vi "多合一臂环解析.vi"(11 "数组":u8[](array[numeric])) -> (0 "chn6":i32(graph), 1 "chn3":i32(graph), 2 "chn8":i32(graph), 3 "chn1":i32(graph), 4 "chn7":i32(graph), 5 "chn2":i32(graph), 6 "chn4":i32(graph), 7 "chn5":i32(graph))   [LabVIEW 2023]
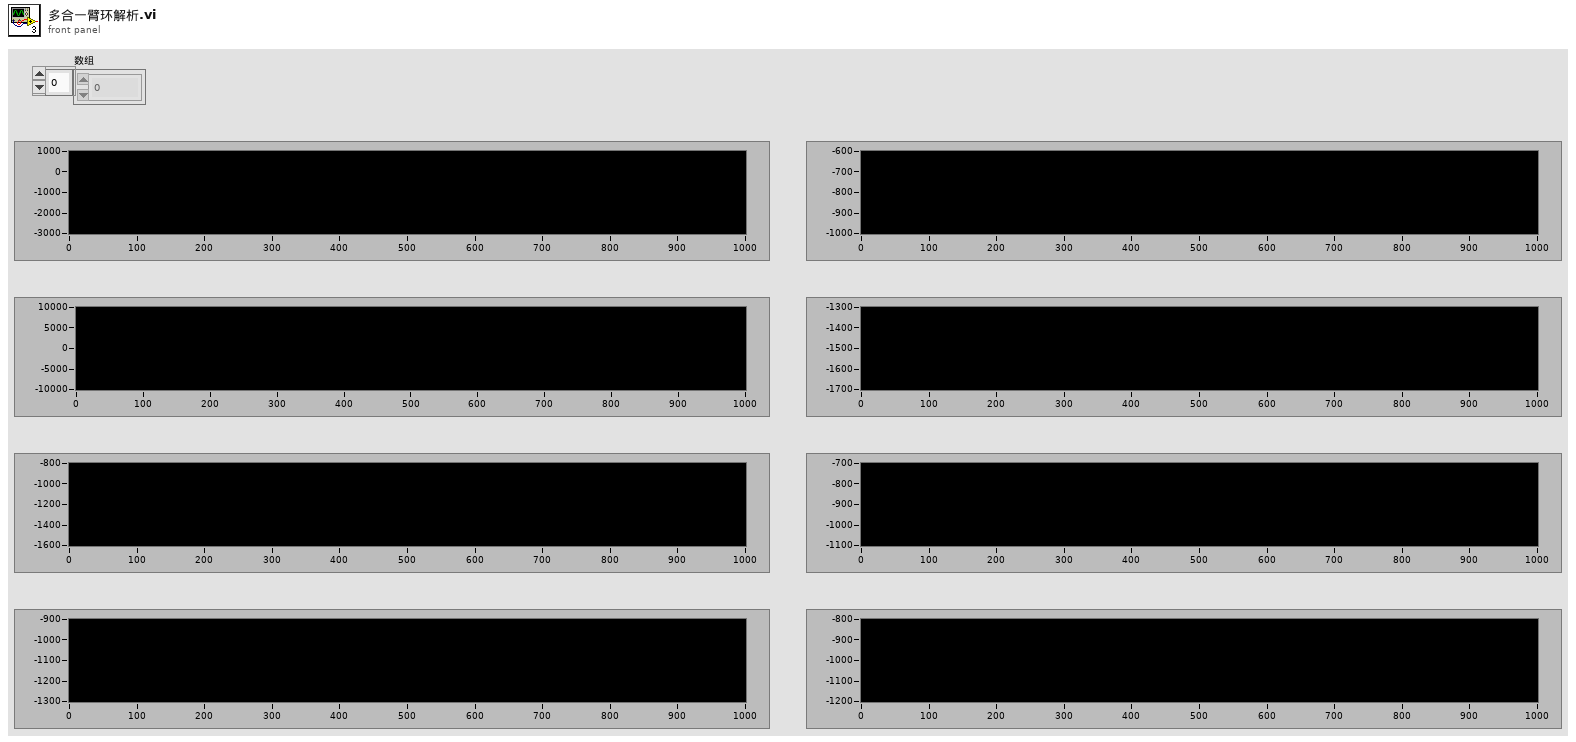
[diagram p1: front panel]
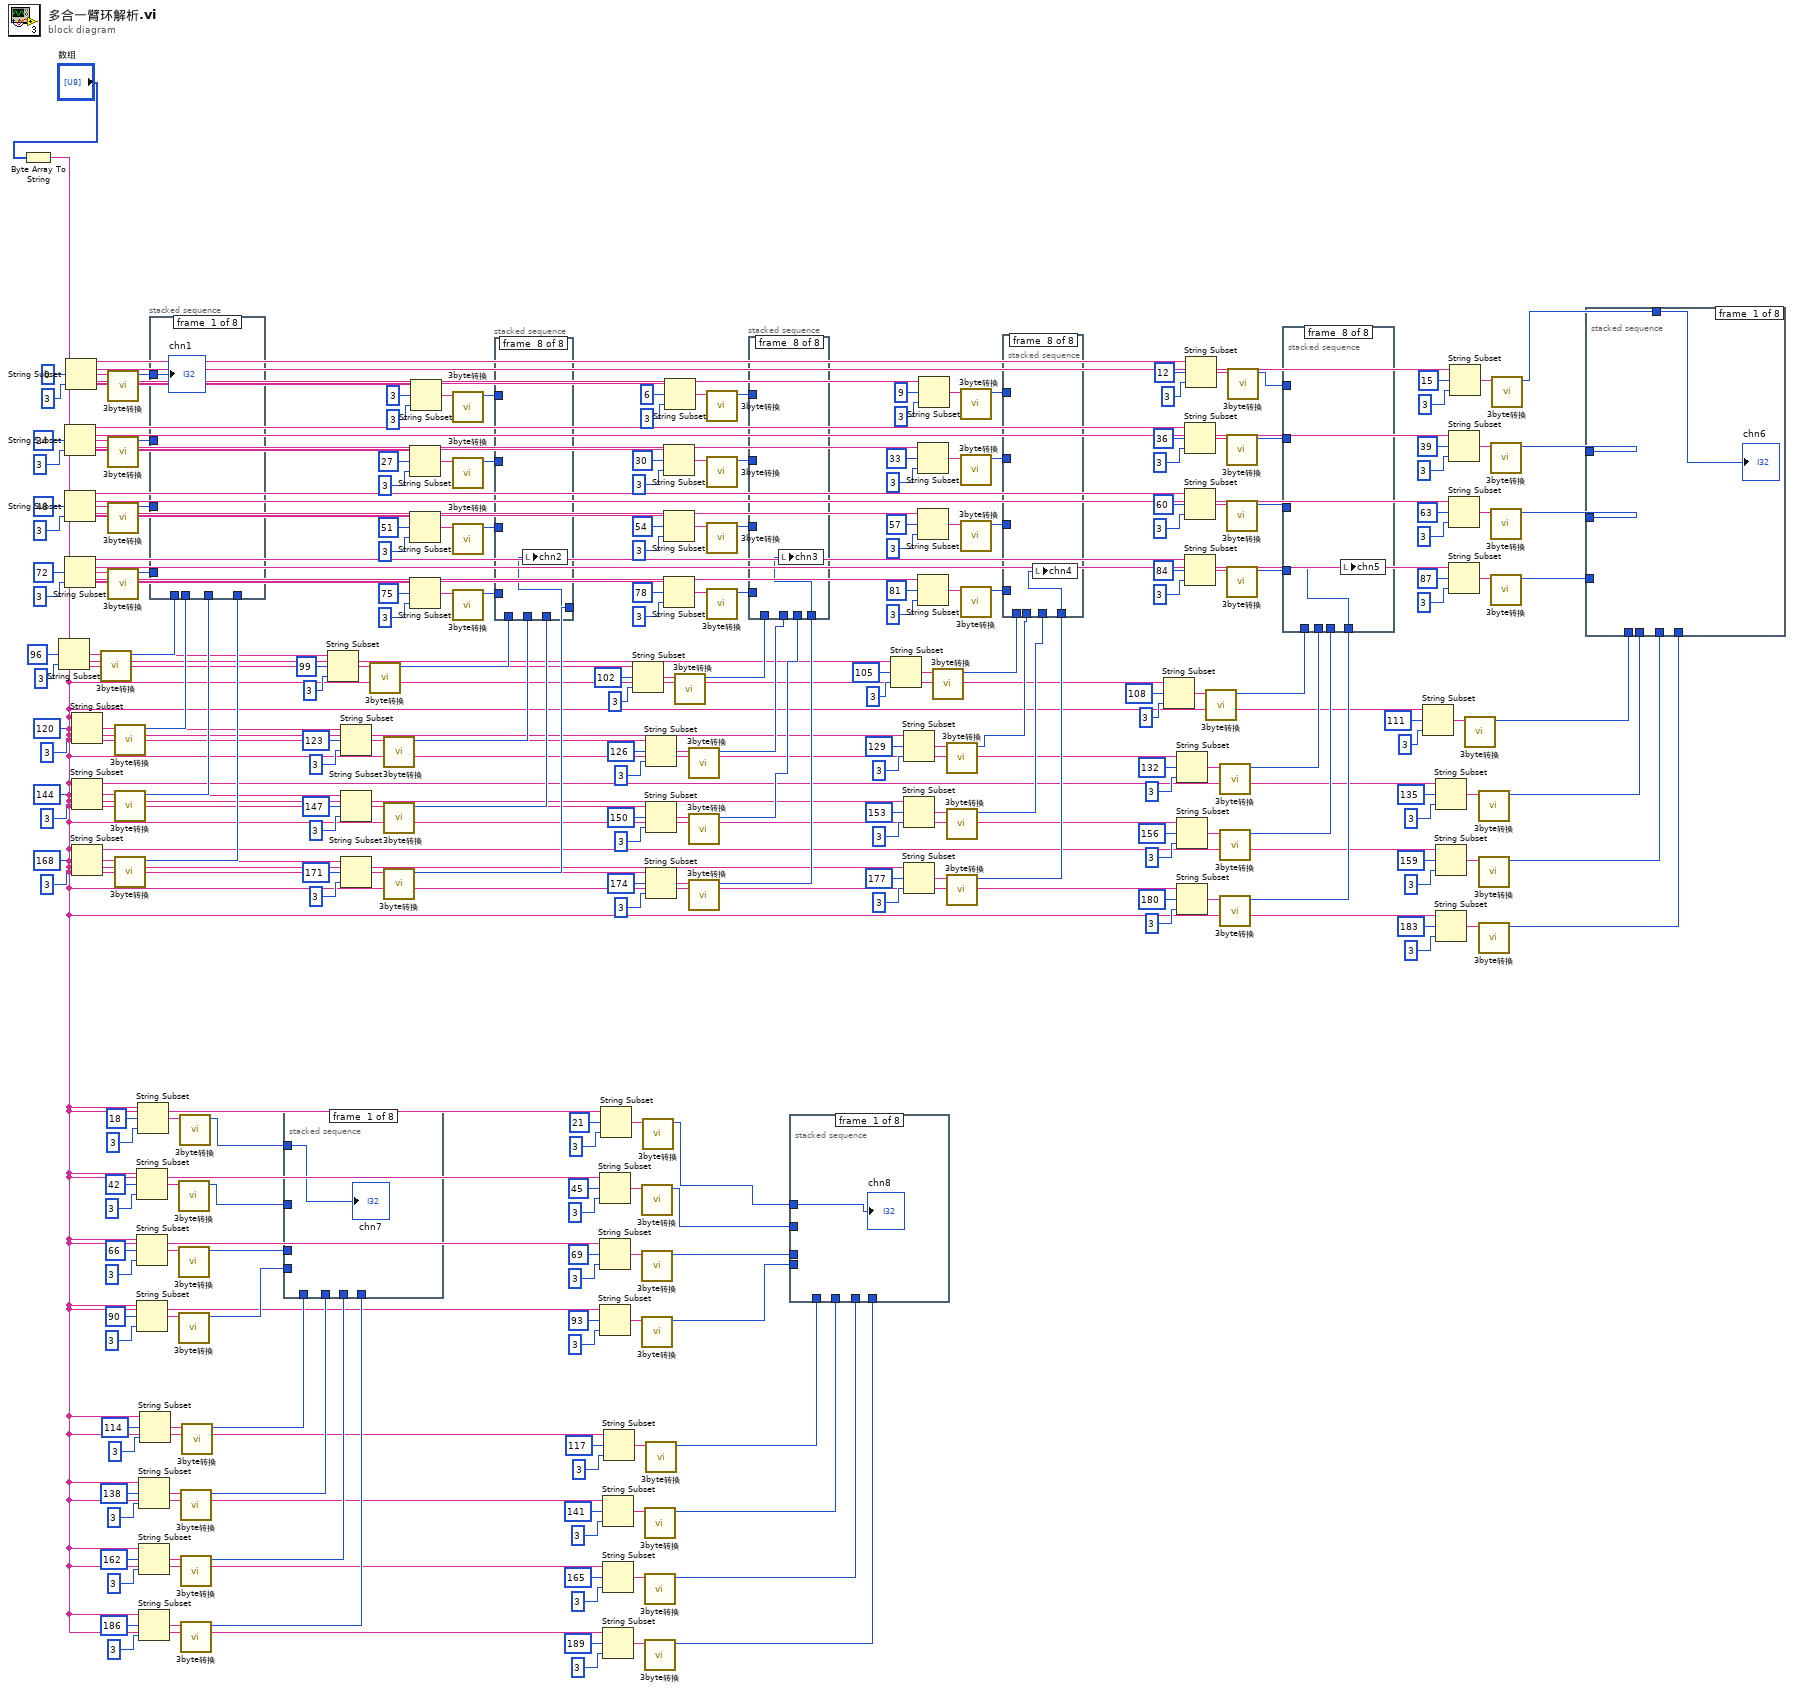
[diagram p0: block diagram]
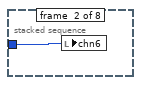
[diagram p2: hidden frame]
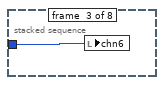
[diagram p3: hidden frame]
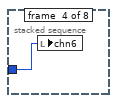
[diagram p4: hidden frame]
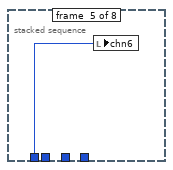
[diagram p5: hidden frame]
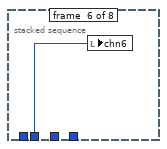
[diagram p6: hidden frame]
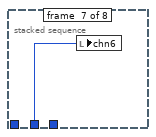
[diagram p7: hidden frame]
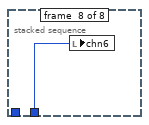
[diagram p8: hidden frame]
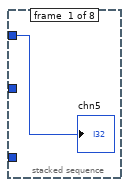
[diagram p9: hidden frame]
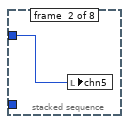
[diagram p10: hidden frame]
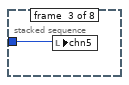
[diagram p11: hidden frame]
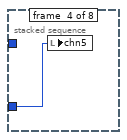
[diagram p12: hidden frame]
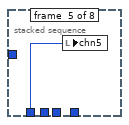
[diagram p13: hidden frame]
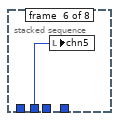
[diagram p14: hidden frame]
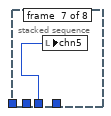
[diagram p15: hidden frame]
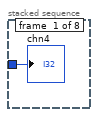
[diagram p16: hidden frame]
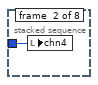
[diagram p17: hidden frame]
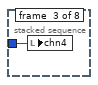
[diagram p18: hidden frame]
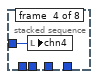
[diagram p19: hidden frame]
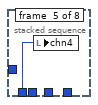
[diagram p20: hidden frame]
diagram:
  n1 = Byte Array To String(unsigned byte array="数组") -> (string=w5:string)
  n2 = String Subset(string=w5, offset (0)=96 ("偏移量(0)"), length (rest)=3 ("长度（剩余）")) -> (substring=w129:string)
  n3 = String Subset(string=w5, offset (0)=24 ("偏移量(0)"), length (rest)=3 ("长度（剩余）")) -> (substring=w256:string)
  n4 = String Subset(string=w5, offset (0)=48 ("偏移量(0)"), length (rest)=3 ("长度（剩余）")) -> (substring=w255:string)
  n5 = String Subset(string=w5, offset (0)=72 ("偏移量(0)"), length (rest)=3 ("长度（剩余）")) -> (substring=w254:string)
  n6 = String Subset(string=w5, offset (0)=0 ("偏移量(0)"), length (rest)=3 ("长度（剩余）")) -> (substring=w257:string)
  n7 = String Subset(string=w5, offset (0)=120 ("偏移量(0)"), length (rest)=3 ("长度（剩余）")) -> (substring=w128:string)
  n8 = String Subset(string=w5, offset (0)=144 ("偏移量(0)"), length (rest)=3 ("长度（剩余）")) -> (substring=w127:string)
  n9 = String Subset(string=w5, offset (0)=168 ("偏移量(0)"), length (rest)=3 ("长度（剩余）")) -> (substring=w126:string)
  n10 = call "3byte转换.vi"("字符串"=w129) -> ("数值"=w118:i32)  [unwired: 10 in]
  n11 = call "3byte转换.vi"("字符串"=w257) -> ("数值"=w245:i32)  [unwired: 10 in]
  n12 = call "3byte转换.vi"("字符串"=w256) -> ("数值"=w244:i32)  [unwired: 10 in]
  n13 = call "3byte转换.vi"("字符串"=w255) -> ("数值"=w243:i32)  [unwired: 10 in]
  n14 = call "3byte转换.vi"("字符串"=w254) -> ("数值"=w242:i32)  [unwired: 10 in]
  n15 = call "3byte转换.vi"("字符串"=w128) -> ("数值"=w117:i32)  [unwired: 10 in]
  n16 = call "3byte转换.vi"("字符串"=w127) -> ("数值"=w116:i32)  [unwired: 10 in]
  n17 = call "3byte转换.vi"("字符串"=w126) -> ("数值"=w115:i32)  [unwired: 10 in]
  n18 = String Subset(string=w5, offset (0)=42 ("偏移量(0)"), length (rest)=3 ("长度（剩余）")) -> (substring=w160:string)
  n19 = String Subset(string=w5, offset (0)=66 ("偏移量(0)"), length (rest)=3 ("长度（剩余）")) -> (substring=w159:string)
  n20 = String Subset(string=w5, offset (0)=90 ("偏移量(0)"), length (rest)=3 ("长度（剩余）")) -> (substring=w158:string)
  n21 = String Subset(string=w5, offset (0)=18 ("偏移量(0)"), length (rest)=3 ("长度（剩余）")) -> (substring=w161:string)
  n22 = String Subset(string=w5, offset (0)=138 ("偏移量(0)"), length (rest)=3 ("长度（剩余）")) -> (substring=w24:string)
  n23 = String Subset(string=w5, offset (0)=162 ("偏移量(0)"), length (rest)=3 ("长度（剩余）")) -> (substring=w25:string)
  n24 = String Subset(string=w5, offset (0)=186 ("偏移量(0)"), length (rest)=3 ("长度（剩余）")) -> (substring=w26:string)
  n25 = String Subset(string=w5, offset (0)=114 ("偏移量(0)"), length (rest)=3 ("长度（剩余）")) -> (substring=w23:string)
  n26 = stacked-sequence {
    tunnel: w245 -> [w259 _ _ _ _ _ _ _]
    tunnel: w244 -> [_ w260 _ _ _ _ _ _]
    tunnel: w243 -> [_ _ w261 _ _ _ _ _]
    tunnel: w242 -> [_ _ _ w262 _ _ _ _]
    tunnel: w118 -> [_ _ _ _ w263 _ _ _]
    tunnel: w117 -> [_ _ _ _ _ w264 _ _]
    tunnel: w116 -> [_ _ _ _ _ _ w265 _]
    tunnel: w115 -> [_ _ _ _ _ _ _ w266]
    frame #0 {
      "chn1" <- w259
    }
    frame #1 {
      n27 = local write "chn1"(w260) -> ()
    }
    frame #2 {
      n28 = local write "chn1"(w261) -> ()
    }
    frame #3 {
      n29 = local write "chn1"(w262) -> ()
    }
    frame #4 {
      n30 = local write "chn1"(w263) -> ()
    }
    frame #5 {
      n31 = local write "chn1"(w264) -> ()
    }
    frame #6 {
      n32 = local write "chn1"(w265) -> ()
    }
    frame #7 {
      n33 = local write "chn1"(w266) -> ()
    }
  }
  n34 = call "3byte转换.vi"("字符串"=w160) -> ("数值"=w149:i32)  [unwired: 10 in]
  n35 = call "3byte转换.vi"("字符串"=w159) -> ("数值"=w148:i32)  [unwired: 10 in]
  n36 = call "3byte转换.vi"("字符串"=w158) -> ("数值"=w147:i32)  [unwired: 10 in]
  n37 = call "3byte转换.vi"("字符串"=w161) -> ("数值"=w150:i32)  [unwired: 10 in]
  n38 = call "3byte转换.vi"("字符串"=w24) -> ("数值"=w20:i32)  [unwired: 10 in]
  n39 = call "3byte转换.vi"("字符串"=w25) -> ("数值"=w19:i32)  [unwired: 10 in]
  n40 = call "3byte转换.vi"("字符串"=w26) -> ("数值"=w18:i32)  [unwired: 10 in]
  n41 = call "3byte转换.vi"("字符串"=w23) -> ("数值"=w21:i32)  [unwired: 10 in]
  n42 = stacked-sequence {
    tunnel: w150 -> [w267 _ _ _ _ _ _ _]
    tunnel: w149 -> [_ w268 _ _ _ _ _ _]
    tunnel: w148 -> [_ _ w269 _ _ _ _ _]
    tunnel: w147 -> [_ _ _ w270 _ _ _ _]
    tunnel: w21 -> [_ _ _ _ w271 _ _ _]
    tunnel: w20 -> [_ _ _ _ _ w272 _ _]
    tunnel: w19 -> [_ _ _ _ _ _ w273 _]
    tunnel: w18 -> [_ _ _ _ _ _ _ w274]
    frame #0 {
      "chn7" <- w267
    }
    frame #1 {
      n43 = local write "chn7"(w268) -> ()
    }
    frame #2 {
      n44 = local write "chn7"(w269) -> ()
    }
    frame #3 {
      n45 = local write "chn7"(w270) -> ()
    }
    frame #4 {
      n46 = local write "chn7"(w271) -> ()
    }
    frame #5 {
      n47 = local write "chn7"(w272) -> ()
    }
    frame #6 {
      n48 = local write "chn7"(w273) -> ()
    }
    frame #7 {
      n49 = local write "chn7"(w274) -> ()
    }
  }
  n50 = String Subset(string=w5, offset (0)=99 ("偏移量(0)"), length (rest)=3 ("长度（剩余）")) -> (substring=w104:string)
  n51 = String Subset(string=w5, offset (0)=123 ("偏移量(0)"), length (rest)=3 ("长度（剩余）")) -> (substring=w105:string)
  n52 = String Subset(string=w5, offset (0)=147 ("偏移量(0)"), length (rest)=3 ("长度（剩余）")) -> (substring=w106:string)
  n53 = String Subset(string=w5, offset (0)=171 ("偏移量(0)"), length (rest)=3 ("长度（剩余）")) -> (substring=w107:string)
  n54 = call "3byte转换.vi"("字符串"=w104) -> ("数值"=w102:i32)  [unwired: 10 in]
  n55 = call "3byte转换.vi"("字符串"=w105) -> ("数值"=w101:i32)  [unwired: 10 in]
  n56 = call "3byte转换.vi"("字符串"=w106) -> ("数值"=w100:i32)  [unwired: 10 in]
  n57 = call "3byte转换.vi"("字符串"=w107) -> ("数值"=w99:i32)  [unwired: 10 in]
  n58 = String Subset(string=w5, offset (0)=27 ("偏移量(0)"), length (rest)=3 ("长度（剩余）")) -> (substring=w232:string)
  n59 = String Subset(string=w5, offset (0)=51 ("偏移量(0)"), length (rest)=3 ("长度（剩余）")) -> (substring=w233:string)
  n60 = String Subset(string=w5, offset (0)=75 ("偏移量(0)"), length (rest)=3 ("长度（剩余）")) -> (substring=w234:string)
  n61 = String Subset(string=w5, offset (0)=3 ("偏移量(0)"), length (rest)=3 ("长度（剩余）")) -> (substring=w231:string)
  n62 = call "3byte转换.vi"("字符串"=w231) -> ("数值"=w229:i32)  [unwired: 10 in]
  n63 = call "3byte转换.vi"("字符串"=w232) -> ("数值"=w228:i32)  [unwired: 10 in]
  n64 = call "3byte转换.vi"("字符串"=w233) -> ("数值"=w227:i32)  [unwired: 10 in]
  n65 = call "3byte转换.vi"("字符串"=w234) -> ("数值"=w226:i32)  [unwired: 10 in]
  n66 = stacked-sequence {
    tunnel: w229 -> [w275 _ _ _ _ _ _ _]
    tunnel: w228 -> [_ w276 _ _ _ _ _ _]
    tunnel: w227 -> [_ _ w277 _ _ _ _ _]
    tunnel: w226 -> [_ _ _ w278 _ _ _ _]
    tunnel: w102 -> [_ _ _ _ w279 _ _ _]
    tunnel: w101 -> [_ _ _ _ _ w280 _ _]
    tunnel: w100 -> [_ _ _ _ _ _ w281 _]
    tunnel: w99 -> [_ _ _ _ _ _ _ w282]
    frame #0 {
      "chn2" <- w275
    }
    frame #1 {
      n67 = local write "chn2"(w276) -> ()
    }
    frame #2 {
      n68 = local write "chn2"(w277) -> ()
    }
    frame #3 {
      n69 = local write "chn2"(w278) -> ()
    }
    frame #4 {
      n70 = local write "chn2"(w279) -> ()
    }
    frame #5 {
      n71 = local write "chn2"(w280) -> ()
    }
    frame #6 {
      n72 = local write "chn2"(w281) -> ()
    }
    frame #7 {
      n73 = local write "chn2"(w282) -> ()
    }
  }
  n74 = String Subset(string=w5, offset (0)=45 ("偏移量(0)"), length (rest)=3 ("长度（剩余）")) -> (substring=w137:string)
  n75 = String Subset(string=w5, offset (0)=69 ("偏移量(0)"), length (rest)=3 ("长度（剩余）")) -> (substring=w138:string)
  n76 = String Subset(string=w5, offset (0)=93 ("偏移量(0)"), length (rest)=3 ("长度（剩余）")) -> (substring=w139:string)
  n77 = String Subset(string=w5, offset (0)=21 ("偏移量(0)"), length (rest)=3 ("长度（剩余）")) -> (substring=w136:string)
  n78 = String Subset(string=w5, offset (0)=141 ("偏移量(0)"), length (rest)=3 ("长度（剩余）")) -> (substring=w15:string)
  n79 = String Subset(string=w5, offset (0)=165 ("偏移量(0)"), length (rest)=3 ("长度（剩余）")) -> (substring=w14:string)
  n80 = String Subset(string=w5, offset (0)=189 ("偏移量(0)"), length (rest)=3 ("长度（剩余）")) -> (substring=w13:string)
  n81 = String Subset(string=w5, offset (0)=117 ("偏移量(0)"), length (rest)=3 ("长度（剩余）")) -> (substring=w16:string)
  n82 = String Subset(string=w5, offset (0)=102 ("偏移量(0)"), length (rest)=3 ("长度（剩余）")) -> (substring=w97:string)
  n83 = call "3byte转换.vi"("字符串"=w137) -> ("数值"=w133:i32)  [unwired: 10 in]
  n84 = call "3byte转换.vi"("字符串"=w138) -> ("数值"=w132:i32)  [unwired: 10 in]
  n85 = call "3byte转换.vi"("字符串"=w139) -> ("数值"=w131:i32)  [unwired: 10 in]
  n86 = call "3byte转换.vi"("字符串"=w136) -> ("数值"=w134:i32)  [unwired: 10 in]
  n87 = call "3byte转换.vi"("字符串"=w15) -> ("数值"=w3:i32)  [unwired: 10 in]
  n88 = call "3byte转换.vi"("字符串"=w14) -> ("数值"=w2:i32)  [unwired: 10 in]
  n89 = call "3byte转换.vi"("字符串"=w13) -> ("数值"=w1:i32)  [unwired: 10 in]
  n90 = String Subset(string=w5, offset (0)=126 ("偏移量(0)"), length (rest)=3 ("长度（剩余）")) -> (substring=w96:string)
  n91 = String Subset(string=w5, offset (0)=150 ("偏移量(0)"), length (rest)=3 ("长度（剩余）")) -> (substring=w95:string)
  n92 = String Subset(string=w5, offset (0)=174 ("偏移量(0)"), length (rest)=3 ("长度（剩余）")) -> (substring=w94:string)
  n93 = call "3byte转换.vi"("字符串"=w16) -> ("数值"=w4:i32)  [unwired: 10 in]
  n94 = String Subset(string=w5, offset (0)=30 ("偏移量(0)"), length (rest)=3 ("长度（剩余）")) -> (substring=w223:string)
  n95 = String Subset(string=w5, offset (0)=54 ("偏移量(0)"), length (rest)=3 ("长度（剩余）")) -> (substring=w222:string)
  n96 = String Subset(string=w5, offset (0)=78 ("偏移量(0)"), length (rest)=3 ("长度（剩余）")) -> (substring=w221:string)
  n97 = String Subset(string=w5, offset (0)=6 ("偏移量(0)"), length (rest)=3 ("长度（剩余）")) -> (substring=w224:string)
  n98 = call "3byte转换.vi"("字符串"=w97) -> ("数值"=w86:i32)  [unwired: 10 in]
  n99 = call "3byte转换.vi"("字符串"=w96) -> ("数值"=w85:i32)  [unwired: 10 in]
  n100 = call "3byte转换.vi"("字符串"=w95) -> ("数值"=w84:i32)  [unwired: 10 in]
  n101 = call "3byte转换.vi"("字符串"=w94) -> ("数值"=w83:i32)  [unwired: 10 in]
  n102 = call "3byte转换.vi"("字符串"=w224) -> ("数值"=w213:i32)  [unwired: 10 in]
  n103 = call "3byte转换.vi"("字符串"=w223) -> ("数值"=w212:i32)  [unwired: 10 in]
  n104 = call "3byte转换.vi"("字符串"=w222) -> ("数值"=w211:i32)  [unwired: 10 in]
  n105 = call "3byte转换.vi"("字符串"=w221) -> ("数值"=w210:i32)  [unwired: 10 in]
  n106 = stacked-sequence {
    tunnel: w213 -> [w283 _ _ _ _ _ _ _]
    tunnel: w212 -> [_ w284 _ _ _ _ _ _]
    tunnel: w211 -> [_ _ w285 _ _ _ _ _]
    tunnel: w210 -> [_ _ _ w286 _ _ _ _]
    tunnel: w86 -> [_ _ _ _ w287 _ _ _]
    tunnel: w85 -> [_ _ _ _ _ w288 _ _]
    tunnel: w84 -> [_ _ _ _ _ _ w289 _]
    tunnel: w83 -> [_ _ _ _ _ _ _ w290]
    frame #0 {
      "chn3" <- w283
    }
    frame #1 {
      n107 = local write "chn3"(w284) -> ()
    }
    frame #2 {
      n108 = local write "chn3"(w285) -> ()
    }
    frame #3 {
      n109 = local write "chn3"(w286) -> ()
    }
    frame #4 {
      n110 = local write "chn3"(w287) -> ()
    }
    frame #5 {
      n111 = local write "chn3"(w288) -> ()
    }
    frame #6 {
      n112 = local write "chn3"(w289) -> ()
    }
    frame #7 {
      n113 = local write "chn3"(w290) -> ()
    }
  }
  n114 = stacked-sequence {
    tunnel: w134 -> [w291 _ _ _ _ _ _ _]
    tunnel: w133 -> [_ w292 _ _ _ _ _ _]
    tunnel: w132 -> [_ _ w293 _ _ _ _ _]
    tunnel: w131 -> [_ _ _ w294 _ _ _ _]
    tunnel: w4 -> [_ _ _ _ w295 _ _ _]
    tunnel: w3 -> [_ _ _ _ _ w296 _ _]
    tunnel: w2 -> [_ _ _ _ _ _ w297 _]
    tunnel: w1 -> [_ _ _ _ _ _ _ w298]
    frame #0 {
      "chn8" <- w291
    }
    frame #1 {
      n115 = local write "chn8"(w292) -> ()
    }
    frame #2 {
      n116 = local write "chn8"(w293) -> ()
    }
    frame #3 {
      n117 = local write "chn8"(w294) -> ()
    }
    frame #4 {
      n118 = local write "chn8"(w295) -> ()
    }
    frame #5 {
      n119 = local write "chn8"(w296) -> ()
    }
    frame #6 {
      n120 = local write "chn8"(w297) -> ()
    }
    frame #7 {
      n121 = local write "chn8"(w298) -> ()
    }
  }
  n122 = String Subset(string=w5, offset (0)=105 ("偏移量(0)"), length (rest)=3 ("长度（剩余）")) -> (substring=w72:string)
  n123 = String Subset(string=w5, offset (0)=129 ("偏移量(0)"), length (rest)=3 ("长度（剩余）")) -> (substring=w73:string)
  n124 = String Subset(string=w5, offset (0)=153 ("偏移量(0)"), length (rest)=3 ("长度（剩余）")) -> (substring=w74:string)
  n125 = String Subset(string=w5, offset (0)=177 ("偏移量(0)"), length (rest)=3 ("长度（剩余）")) -> (substring=w75:string)
  n126 = String Subset(string=w5, offset (0)=33 ("偏移量(0)"), length (rest)=3 ("长度（剩余）")) -> (substring=w200:string)
  n127 = String Subset(string=w5, offset (0)=57 ("偏移量(0)"), length (rest)=3 ("长度（剩余）")) -> (substring=w201:string)
  n128 = String Subset(string=w5, offset (0)=81 ("偏移量(0)"), length (rest)=3 ("长度（剩余）")) -> (substring=w202:string)
  n129 = String Subset(string=w5, offset (0)=9 ("偏移量(0)"), length (rest)=3 ("长度（剩余）")) -> (substring=w199:string)
  n130 = call "3byte转换.vi"("字符串"=w72) -> ("数值"=w70:i32)  [unwired: 10 in]
  n131 = call "3byte转换.vi"("字符串"=w73) -> ("数值"=w69:i32)  [unwired: 10 in]
  n132 = call "3byte转换.vi"("字符串"=w74) -> ("数值"=w68:i32)  [unwired: 10 in]
  n133 = call "3byte转换.vi"("字符串"=w75) -> ("数值"=w67:i32)  [unwired: 10 in]
  n134 = call "3byte转换.vi"("字符串"=w199) -> ("数值"=w197:i32)  [unwired: 10 in]
  n135 = call "3byte转换.vi"("字符串"=w200) -> ("数值"=w196:i32)  [unwired: 10 in]
  n136 = call "3byte转换.vi"("字符串"=w201) -> ("数值"=w195:i32)  [unwired: 10 in]
  n137 = call "3byte转换.vi"("字符串"=w202) -> ("数值"=w194:i32)  [unwired: 10 in]
  n138 = stacked-sequence {
    tunnel: w197 -> [w299 _ _ _ _ _ _ _]
    tunnel: w196 -> [_ w300 _ _ _ _ _ _]
    tunnel: w195 -> [_ _ w301 _ _ _ _ _]
    tunnel: w194 -> [_ _ _ w302 _ _ _ _]
    tunnel: w70 -> [_ _ _ _ w303 _ _ _]
    tunnel: w69 -> [_ _ _ _ _ w304 _ _]
    tunnel: w68 -> [_ _ _ _ _ _ w305 _]
    tunnel: w67 -> [_ _ _ _ _ _ _ w306]
    frame #0 {
      "chn4" <- w299
    }
    frame #1 {
      n139 = local write "chn4"(w300) -> ()
    }
    frame #2 {
      n140 = local write "chn4"(w301) -> ()
    }
    frame #3 {
      n141 = local write "chn4"(w302) -> ()
    }
    frame #4 {
      n142 = local write "chn4"(w303) -> ()
    }
    frame #5 {
      n143 = local write "chn4"(w304) -> ()
    }
    frame #6 {
      n144 = local write "chn4"(w305) -> ()
    }
    frame #7 {
      n145 = local write "chn4"(w306) -> ()
    }
  }
  n146 = String Subset(string=w5, offset (0)=108 ("偏移量(0)"), length (rest)=3 ("长度（剩余）")) -> (substring=w65:string)
  n147 = String Subset(string=w5, offset (0)=132 ("偏移量(0)"), length (rest)=3 ("长度（剩余）")) -> (substring=w64:string)
  n148 = String Subset(string=w5, offset (0)=156 ("偏移量(0)"), length (rest)=3 ("长度（剩余）")) -> (substring=w63:string)
  n149 = String Subset(string=w5, offset (0)=180 ("偏移量(0)"), length (rest)=3 ("长度（剩余）")) -> (substring=w62:string)
  n150 = String Subset(string=w5, offset (0)=36 ("偏移量(0)"), length (rest)=3 ("长度（剩余）")) -> (substring=w191:string)
  n151 = String Subset(string=w5, offset (0)=60 ("偏移量(0)"), length (rest)=3 ("长度（剩余）")) -> (substring=w190:string)
  n152 = String Subset(string=w5, offset (0)=84 ("偏移量(0)"), length (rest)=3 ("长度（剩余）")) -> (substring=w189:string)
  n153 = String Subset(string=w5, offset (0)=12 ("偏移量(0)"), length (rest)=3 ("长度（剩余）")) -> (substring=w192:string)
  n154 = call "3byte转换.vi"("字符串"=w65) -> ("数值"=w54:i32)  [unwired: 10 in]
  n155 = call "3byte转换.vi"("字符串"=w64) -> ("数值"=w53:i32)  [unwired: 10 in]
  n156 = call "3byte转换.vi"("字符串"=w63) -> ("数值"=w52:i32)  [unwired: 10 in]
  n157 = call "3byte转换.vi"("字符串"=w62) -> ("数值"=w51:i32)  [unwired: 10 in]
  n158 = call "3byte转换.vi"("字符串"=w191) -> ("数值"=w180:i32)  [unwired: 10 in]
  n159 = call "3byte转换.vi"("字符串"=w190) -> ("数值"=w179:i32)  [unwired: 10 in]
  n160 = call "3byte转换.vi"("字符串"=w189) -> ("数值"=w178:i32)  [unwired: 10 in]
  n161 = call "3byte转换.vi"("字符串"=w192) -> ("数值"=w181:i32)  [unwired: 10 in]
  n162 = stacked-sequence {
    tunnel: w181 -> [w307 _ _ _ _ _ _ _]
    tunnel: w180 -> [_ w308 _ _ _ _ _ _]
    tunnel: w179 -> [_ _ w309 _ _ _ _ _]
    tunnel: w178 -> [_ _ _ w310 _ _ _ _]
    tunnel: w54 -> [_ _ _ _ w311 _ _ _]
    tunnel: w53 -> [_ _ _ _ _ w312 _ _]
    tunnel: w52 -> [_ _ _ _ _ _ w313 _]
    tunnel: w51 -> [_ _ _ _ _ _ _ w314]
    frame #0 {
      "chn5" <- w307
    }
    frame #1 {
      n163 = local write "chn5"(w308) -> ()
    }
    frame #2 {
      n164 = local write "chn5"(w309) -> ()
    }
    frame #3 {
      n165 = local write "chn5"(w310) -> ()
    }
    frame #4 {
      n166 = local write "chn5"(w311) -> ()
    }
    frame #5 {
      n167 = local write "chn5"(w312) -> ()
    }
    frame #6 {
      n168 = local write "chn5"(w313) -> ()
    }
    frame #7 {
      n169 = local write "chn5"(w314) -> ()
    }
  }
  n170 = String Subset(string=w5, offset (0)=111 ("偏移量(0)"), length (rest)=3 ("长度（剩余）")) -> (substring=w39:string)
  n171 = String Subset(string=w5, offset (0)=135 ("偏移量(0)"), length (rest)=3 ("长度（剩余）")) -> (substring=w40:string)
  n172 = String Subset(string=w5, offset (0)=159 ("偏移量(0)"), length (rest)=3 ("长度（剩余）")) -> (substring=w41:string)
  n173 = String Subset(string=w5, offset (0)=183 ("偏移量(0)"), length (rest)=3 ("长度（剩余）")) -> (substring=w42:string)
  n174 = String Subset(string=w5, offset (0)=39 ("偏移量(0)"), length (rest)=3 ("长度（剩余）")) -> (substring=w168:string)
  n175 = String Subset(string=w5, offset (0)=63 ("偏移量(0)"), length (rest)=3 ("长度（剩余）")) -> (substring=w169:string)
  n176 = String Subset(string=w5, offset (0)=87 ("偏移量(0)"), length (rest)=3 ("长度（剩余）")) -> (substring=w170:string)
  n177 = String Subset(string=w5, offset (0)=15 ("偏移量(0)"), length (rest)=3 ("长度（剩余）")) -> (substring=w167:string)
  n178 = call "3byte转换.vi"("字符串"=w39) -> ("数值"=w37:i32)  [unwired: 10 in]
  n179 = call "3byte转换.vi"("字符串"=w40) -> ("数值"=w36:i32)  [unwired: 10 in]
  n180 = call "3byte转换.vi"("字符串"=w41) -> ("数值"=w35:i32)  [unwired: 10 in]
  n181 = call "3byte转换.vi"("字符串"=w42) -> ("数值"=w34:i32)  [unwired: 10 in]
  n182 = call "3byte转换.vi"("字符串"=w168) -> ("数值"=w164:i32)  [unwired: 10 in]
  n183 = call "3byte转换.vi"("字符串"=w169) -> ("数值"=w163:i32)  [unwired: 10 in]
  n184 = call "3byte转换.vi"("字符串"=w170) -> ("数值"=w50:i32)  [unwired: 10 in]
  n185 = call "3byte转换.vi"("字符串"=w167) -> ("数值"=w165:i32)  [unwired: 10 in]
  n186 = stacked-sequence {
    tunnel: w165 -> [w315 _ _ _ _ _ _ _]
    tunnel: w164 -> [_ w316 _ _ _ _ _ _]
    tunnel: w163 -> [_ _ w317 _ _ _ _ _]
    tunnel: w50 -> [_ _ _ w318 _ _ _ _]
    tunnel: w37 -> [_ _ _ _ w319 _ _ _]
    tunnel: w36 -> [_ _ _ _ _ w320 _ _]
    tunnel: w35 -> [_ _ _ _ _ _ w321 _]
    tunnel: w34 -> [_ _ _ _ _ _ _ w322]
    frame #0 {
      "chn6" <- w315
    }
    frame #1 {
      n187 = local write "chn6"(w316) -> ()
    }
    frame #2 {
      n188 = local write "chn6"(w317) -> ()
    }
    frame #3 {
      n189 = local write "chn6"(w318) -> ()
    }
    frame #4 {
      n190 = local write "chn6"(w319) -> ()
    }
    frame #5 {
      n191 = local write "chn6"(w320) -> ()
    }
    frame #6 {
      n192 = local write "chn6"(w321) -> ()
    }
    frame #7 {
      n193 = local write "chn6"(w322) -> ()
    }
  }
